vi "rebuildMessage.vi"(0 "Host_Reference":refnum<class "HGF_Reference.lvclass">, 2 "Object Data":string, 5 "error in (no error)":errorcluster) -> (14 "dup HGF_Reference":refnum<class "HGF_Reference.lvclass">, 16 "MoAgSy_Message":refnum<class "MoAgSy_Message.lvclass">, 19 "error out":errorcluster)   [LabVIEW 2009, in "MoAgSy.lvlib" / "MoAgSy_Host.lvclass"]
uses:
  MoAgSy_Host.lvclass
  HGF_BaseClasses/HGF_Reference/HGF_Reference.lvclass
  MoAgSy_Message/MoAgSy_Message.lvclass
panel:
  in  "TEST?":bool
  in  "timeout in ms (-1)":i32=-1
  out "Class Path":path
  out "Object":string
  out "Class":string
  out "Library":string
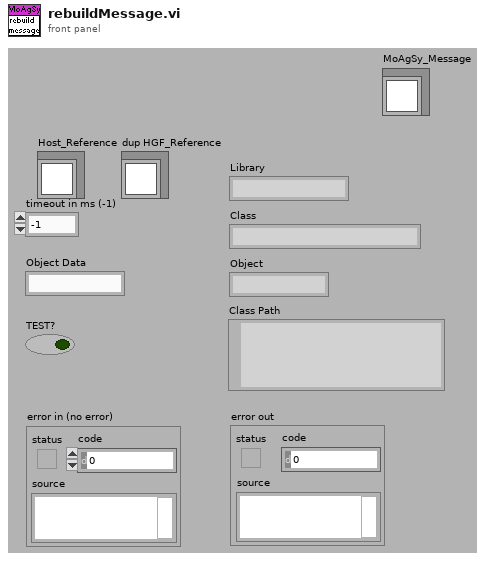
[diagram p1: front panel]
types:
  T1 = cluster{"Working Folder":path, "Class Folder":path}
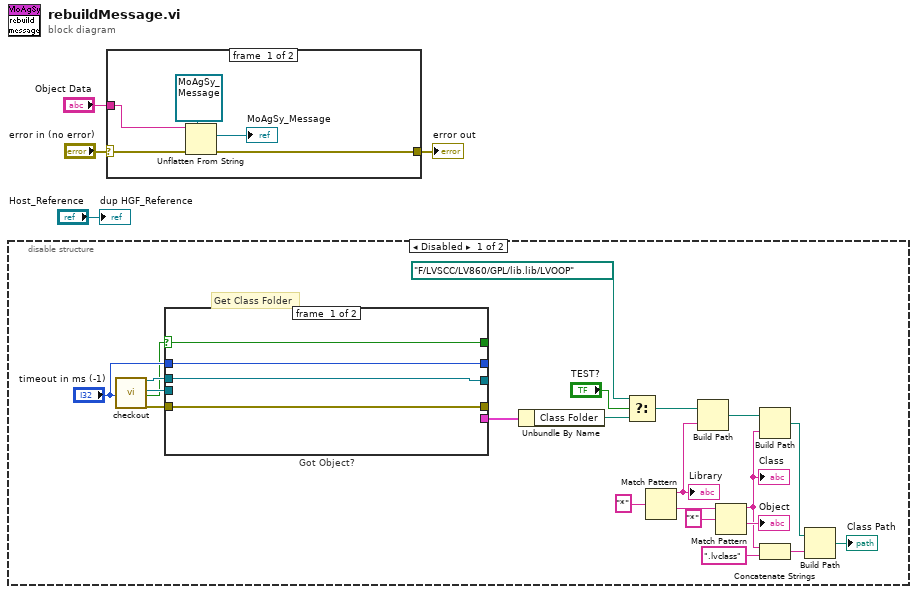
[diagram p0: block diagram]
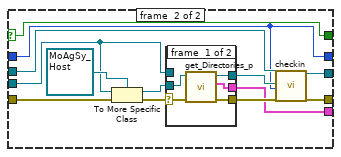
[diagram p2: hidden frame]
diagram:
  n1 = disable-structure shown="Disabled" {
    frame #0 {
      # "Get Class Folder"
      n2 = call "checkout.vi"("timeout in ms (-1)"="timeout in ms (-1)") -> ("dup HGF_Reference"=w19:refnum<class "HGF_Reference.lvclass">, "Object"=w18:refnum<class>, "got object?"=w17:bool, "error out"=w16:errorcluster)  [unwired: 2 in, 13 out]
      n3 = case "Got Object?" shown="True" w17 {
        selector: w17 -> [w26 w33]
        tunnel: w18 -> [_ w30]
        tunnel: w19 -> [w29 w42]
        tunnel: [w29 w41] -> _
        tunnel: "timeout in ms (-1)" -> [w27 w34]
        tunnel: [w28 w40] -> _
        tunnel: w16 -> [w28 w39]
        tunnel: [_ w36] -> w21
        tunnel: [w27 w34] -> _
        tunnel: [w26 w33] -> _
        frame #0 {
        }
        frame #1 {
          n4 = To More Specific Class(target class=refnum<class "MoAgSy_Host.lvclass"> refnum ("MoAgSy.lvlib:MoAgSy_Host.lvclass"), reference=w30, error in=w39) -> (specific class reference=w35:refnum<class "MoAgSy_Host.lvclass">, error out=w31:errorcluster)
          n5 = case shown="No Error" w31 {
            selector: w31 -> [w43 w48]
            tunnel: [w46 w49] -> w38
            tunnel: [w44 w48] -> w37
            tunnel: [w45 _] -> w36
            tunnel: w35 -> [w47 _]
            tunnel: w30 -> [_ w49]
            frame #0 {
              n6 = call "get_Directories_p.vi"("error in (no error)"=w43, "MoAgSy_Host in"=w47) -> ("error out"=w44:errorcluster, "Directories"=w45:T1, "MoAgSy_Host out"=w46:refnum<class "MoAgSy_Host.lvclass">)  [unwired: 7 out]
            }
            frame #1 {
            }
          }
          n7 = call "checkin.vi"("HGF_Reference"=w42, "Object"=w38, "timeout /ms (-1)"=w34, "error in (no error)"=w37) -> ("dup HGF_Reference"=w41:refnum<class "HGF_Reference.lvclass">, "error out"=w40:errorcluster)  [unwired: 14 out]
        }
      }
      n8 = Unbundle By Name(w21) -> ("Class Folder"=w24:path)
      n9 = Select(t=path "F:/LVSCC/LV860/GPL/lib.lib/LVOOP", s="TEST?", f=w24) -> (s? t:f=w25:path)
      n10 = Match Pattern(regular expression="*") -> (before substring=w8:string, after substring=w7:string)  [unwired: 1 in, 3 out]
      "Library" <- w8
      n11 = Build Path(base path=w25, name or relative path=w8) -> (appended path=w9:path)
      n12 = Match Pattern(string=w7, regular expression="*") -> (before substring=w10:string, after substring=→"Object":string)  [unwired: 3 out]
      "Class" <- w10
      n13 = Build Path(base path=w9, name or relative path=w10) -> (appended path=w13:path)
      n14 = Concatenate Strings(w10, ".lvclass" ("string")) -> (w12:string)
      n15 = Build Path(base path=w13, name or relative path=w12) -> (appended path=→"Class Path":path)
    }
    frame #1 {
    }
  }
  n16 = case shown="No Error" "error in (no error)" {
    selector: "error in (no error)" -> [w52 w55]
    tunnel: "Object Data" -> [w53 _]
    tunnel: [w51 w55] -> w4
    frame #0 {
      n17 = Unflatten From String(type=refnum<class "MoAgSy_Message.lvclass"> refnum ("MoAgSy.lvlib:MoAgSy_Message.lvclass"), binary string=w53, error in (no error)=w52) -> (value=→"MoAgSy_Message":refnum<class "MoAgSy_Message.lvclass">, error out=w51:errorcluster)  [unwired: 3 out]
    }
    frame #1 {
    }
  }
  "error out" <- w4
  "dup HGF_Reference" <- "Host_Reference"
